vi "Set Switch.vi"(8 "error in (no error)":errorcluster, 9 "switch name":string="A", 10 "value":bool, 11 "MC switch refnum in":refnum<k24>) -> (0 "error out":errorcluster, 3 "MC switch refnum out":refnum<k24>)   [LabVIEW 2019, in "Minicircuit RF Switch Box.lvlib"]
doc: "This function sets an individual SPDT within the switch matrix while leaving any other switches unchanged.\nThe switches are designated A to H, as labeled on the front of the switch matrix\n\n<b>Note:</b> If the swish matrix does not have a swich connected to the ask position, nothing will append."
uses:
  <instrlib>/LV_Minicircuit_RF_Switch/Minicircuit RF Switch Box.lvlib
  C:/Program Files (x86)/National Instruments/LabVIEW 2019/instr.lib/LV_Minicircuit_RF_Switch/mcl_RF_Switch_Controller_NET45.dll
  mcl_RF_Switch_Controller_NET45.dll
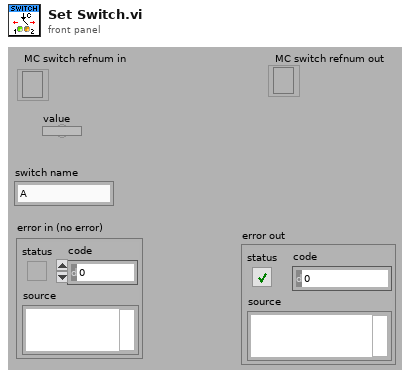
[diagram p1: front panel]
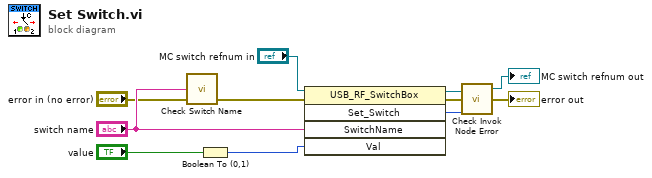
[diagram p0: block diagram]
diagram:
  n1 = call <instrlib>:"Check Switch Name.vi"("error in (no error)"="error in (no error)", "switch name in"="switch name") -> ("error out"=w1:errorcluster)  [unwired: 2 in, 1 out]
  n2 = Boolean To (0,1)(Boolean="value") -> (0, 1=w4:i16)
  n3 = invoke class="USB_RF_SwitchBox" method="Set_Switch"(reference="MC switch refnum in", error in=w1, "SwitchName"="switch name", "Val"=w4) -> (reference out=w10:refnum<k24>, error out=w9:errorcluster, "Set_Switch"=w8:i32)  [unwired: 1 in, 2 out]
  n4 = call <instrlib>:"Check Invok Node Error.vi"("Connect"=w8, "error in (no error)"=w9, "MC switch refnum in"=w10) -> ("error out"=→"error out":errorcluster, "MC switch refnum out"=→"MC switch refnum out":refnum<k24>)  [unwired: 1 in]
